vi "Untitled 3 (SubVI).vi"(4 "NIM":string, 5 "Boolean":bool, 6 "Nama":string, 7 "Foto":path, 8 "error in (no error)":errorcluster, 10 "Email":string, 11 "Refnum in":T1) -> (0 "error out":errorcluster, 2 "resulting string":string, 3 "Refnum out":T1)   [LabVIEW 2024]
uses:
  <vilib>/addons/database/Connection.llb/Conn ObjectReference.ctl
  <vilib>/addons/database/Connection.llb/Conn Execute.vi
  <vilib>/addons/database/NI_Database_API.lvlib
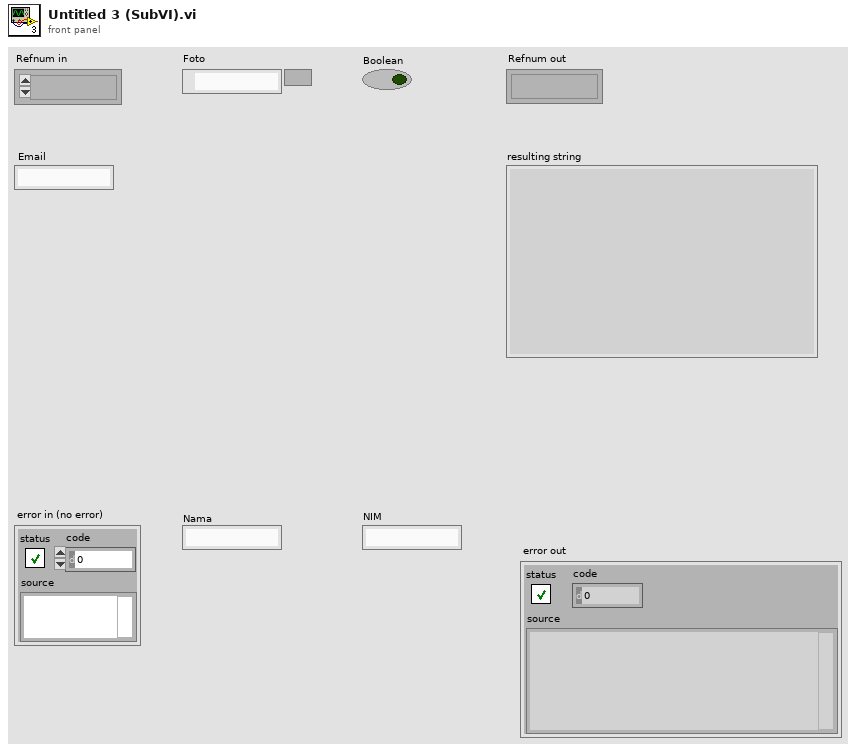
[diagram p1: front panel]
types:
  T1 = typedef "NI_Database_API.lvlib/Conn ObjectReference.ctl" = refnum<k1>
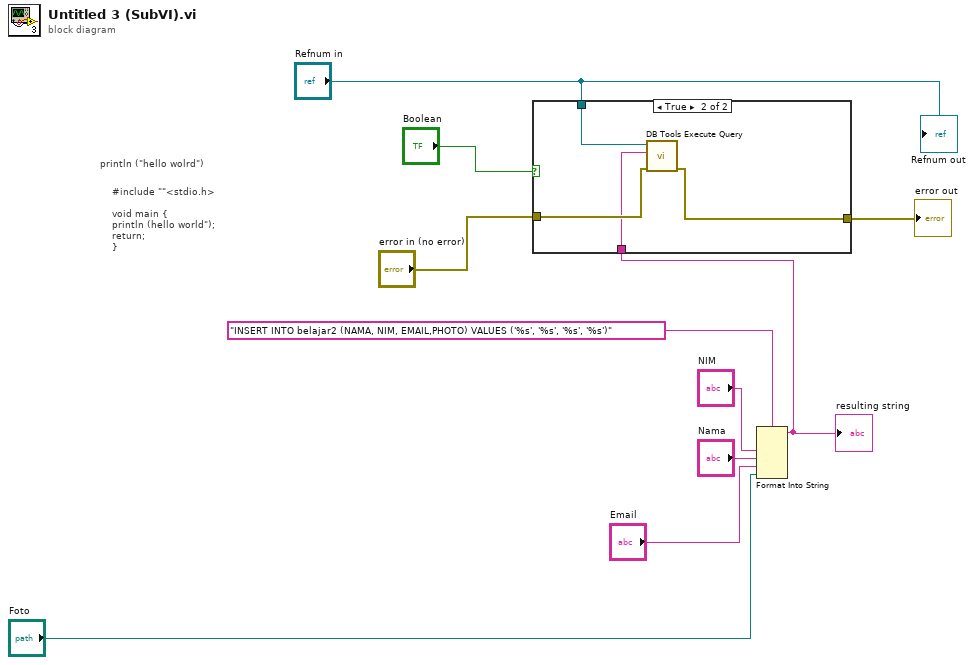
[diagram p0: block diagram]
diagram:
  # "#include \"\"<stdio.h>\n\nvoid main {\nprintln (hello world\");\nreturn;\n}"
  # "println (\"hello wolrd\")"
  n1 = Format Into String(format string="INSERT INTO belajar2 (NAMA, NIM, EMAIL,PHOTO) VALUES ('%s', '%s', '%s', '%s')", "NIM", "Nama", "Email", "Foto") -> (resulting string=w10:string)  [unwired: 2 in, 1 out]
  "resulting string" <- w10
  n2 = case shown="True" "Boolean" {
    tunnel: "Refnum in" -> [_ w15]
    tunnel: "error in (no error)" -> [w11 w14]
    tunnel: [w11 w13] -> w5
    tunnel: w10 -> [_ w12]
    frame False {
    }
    frame True {
      n3 = call-poly <vilib>:"DB Tools Execute Query.vi"("error in (no error)"=w14, "SQL query"=w12, "connection reference"=w15) -> ("error out"=w13:errorcluster)  [unwired: 5 in, 1 out]
    }
  }
  "error out" <- w5
  "Refnum out" <- "Refnum in"
